vi "PDCInitDevice.vi"(8 "error in (no error)":errorcluster, 11 "String":string) -> (0 "error out":errorcluster, 3 "DeviceNo":u32)   [LabVIEW 2015]
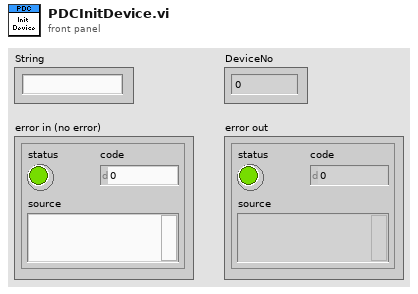
[diagram p1: front panel]
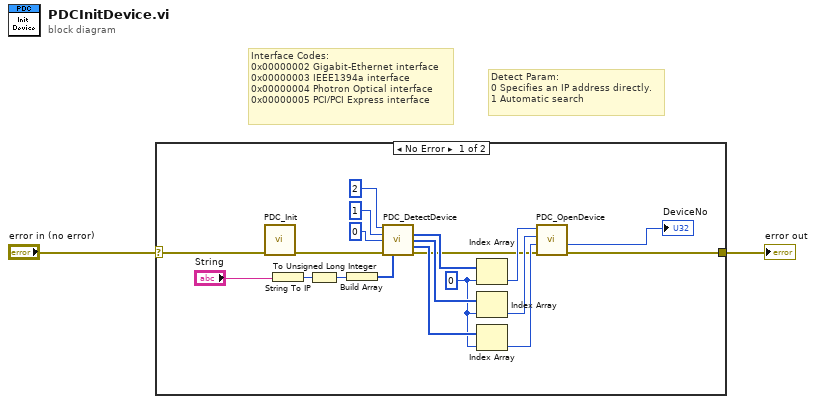
[diagram p0: block diagram]
diagram:
  # "Detect Param:\n0 Specifies an IP address directly.\n1 Automatic search"
  # "Interface Codes:\n0x00000002 Gigabit-Ethernet interface \n0x00000003 IEEE1394a interface \n0x00000004 Photron Optical interface\n0x00000005 PCI/PCI Express interface"
  n1 = case shown="No Error" "error in (no error)" {
    selector: "error in (no error)" -> [w3 w22]
    tunnel: [w20 w22] -> w2
    frame No Error {
      w13 = 0 ("Žw•W")
      n2 = call "PDC_Init.vi"("error in (no error)"=w3) -> ("error out"=w4:errorcluster)  [unwired: 8 in, 2 out]
      n3 = String To IP(1:"String") -> (0:w9:u32)
      n4 = To Unsigned Long Integer(number=w9) -> (unsigned 32bit integer=w10:u32)
      n5 = Build Array(w10) -> (w11:u32[])
      n6 = call "PDC_DetectDevice.vi"("InterfaceCode"=u32 2, "DetectNum"=u32 1, "DetectParam"=u32 0, "error in (no error)"=w4, "DetectNo"=w11) -> ("DeviceCode"=w14:u32[], "TmpDeviceNo"=w15:u32[], "InterfaceCode(out)"=w16:u32[], "error out"=w12:errorcluster)  [unwired: 4 in, 3 out]
      n7 = Index Array(array=w14, index=w13) -> (element=w17:u32)
      n8 = Index Array(array=w15, index=w13) -> (element=w18:u32)
      n9 = Index Array(array=w16, index=w13) -> (element=w19:u32)
      n10 = call "PDC_OpenDevice.vi"("error in (no error)"=w12, "InterfaceCode"=w19, "TmpDeviceNo"=w18, "DeviceCode"=w17) -> ("error out"=w20:errorcluster, "DeviceNo"=→"DeviceNo":u32)  [unwired: 4 in, 2 out]
    }
    frame Error {
    }
  }
  "error out" <- w2
